vi "Set Number Accumulations.vi"(8 "error in (no error)":errorcluster, 11 "number":i32) -> (0 "error out":errorcluster, 3 "function return":u32)   [LabVIEW 2018, in "AndorSDK.lvlib"]
doc: "EXPNETTYPE unsigned int WINAPI SetNumberAccumulations(int number);"
uses:
  AndorSDK.lvlib
  ATMCD32D.dll
  OwnVIs/AndorOWN.lvlib
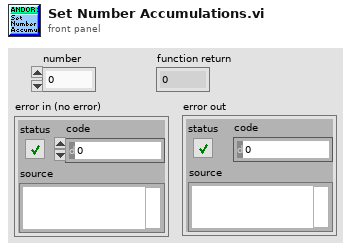
[diagram p1: front panel]
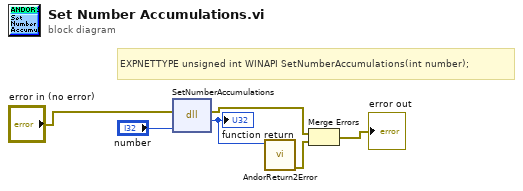
[diagram p0: block diagram]
diagram:
  # "EXPNETTYPE unsigned int WINAPI SetNumberAccumulations(int number);"
  n1 = dll-call lib="C:/Users/johan/Downloads/LabVIEW software/LabVIEW software/IX-81 Software/lib/ANDOR/Andor SDK/ATMCD32D.*" fn="SetNumberAccumulations"(error in="error in (no error)", "number"="number") -> (error out=w4:errorcluster, w5:u32)  [unwired: 3 in, 1 out]
  "function return" <- w5
  n2 = call "AndorReturn2Error.vi"("Camera return"=w5) -> ("error out"=w3:errorcluster)  [unwired: 10 in]
  n3 = Merge Errors(w4, w3) -> (→"error out":errorcluster)
